vi "PathGlobal.vi"(10 "Path":T1=[{"X"=0.0, "Y"=0.0, "OnOff"=TRUE}, {"X"=0.0, "Y"=0.5, "OnOff"=TRUE}, {"X"=0.5, "Y"=1.0, "OnOff"=TRUE}, {"X"=1.0, "Y"=0.5, "OnOff"=TRUE}, {"X"=0.5, "Y"=0.0, "OnOff"=TRUE}, {"X"=0.0, "Y"=0.5, "OnOff"=TRUE}, {"X"=0.0, "Y"=0.0, "OnOff"=TRUE}], 11 "Set/Get":bool) -> (3 "PathOut":T1=[{"X"=0.0, "Y"=0.0, "OnOff"=TRUE}, {"X"=0.0, "Y"=0.5, "OnOff"=TRUE}, {"X"=0.5, "Y"=1.0, "OnOff"=TRUE}, {"X"=1.0, "Y"=0.5, "OnOff"=TRUE}, {"X"=0.5, "Y"=0.0, "OnOff"=TRUE}, {"X"=0.0, "Y"=0.5, "OnOff"=TRUE}, {"X"=0.0, "Y"=0.0, "OnOff"=TRUE}])   [LabVIEW 2014]
uses:
  Path.ctl
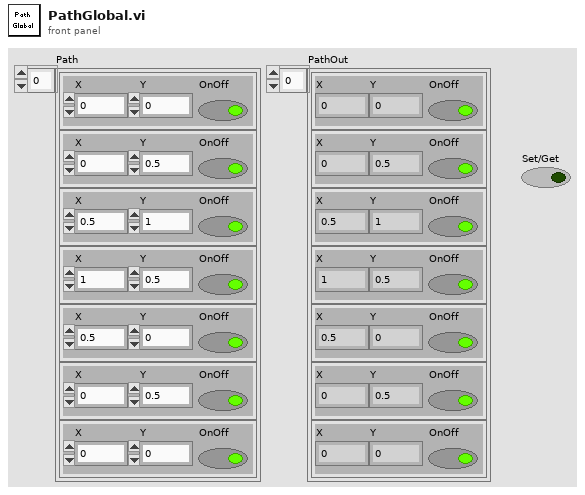
[diagram p1: front panel]
types:
  T1 = typedef "Path.ctl" = cluster{"X":dbl, "Y":dbl, "OnOff":bool}[]
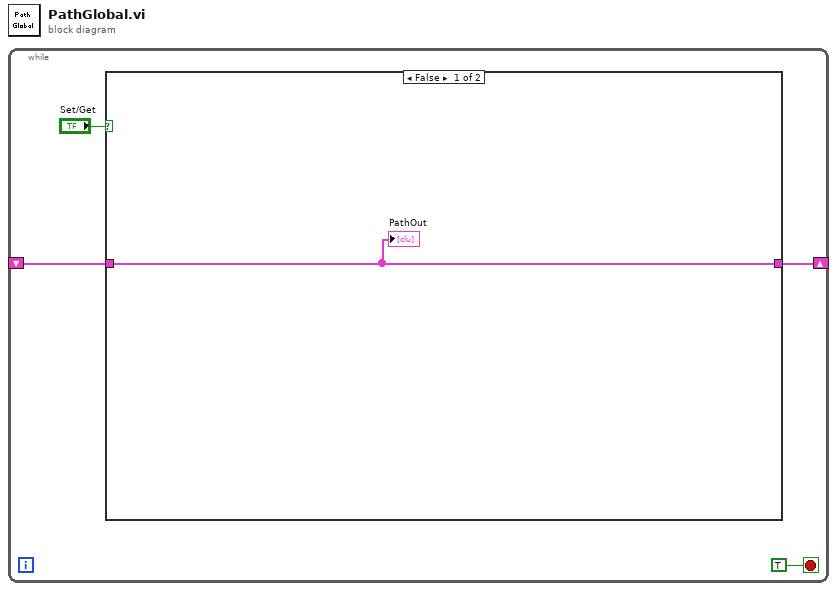
[diagram p0: block diagram]
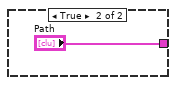
[diagram p2: hidden frame]
diagram:
  n1 = while {
    shift-right: [w2] -> _
    shift-left: _ -> [w1]
    stop <- TRUE stop-if-true
    n2 = case shown="False" "Set/Get" {
      tunnel: [w5 "Path"] -> w2
      tunnel: w1 -> [w5 _]
      frame False {
        "PathOut" <- w5
      }
      frame True {
      }
    }
  }
